vi "Write Current.vi"(8 "error in":errorcluster, 10 "Current":dbl, 11 "69X_79X in":refnum<class "79XRP.lvclass">) -> (0 "error out":errorcluster, 3 "69X_79X out":refnum<class "79XRP.lvclass">)   [LabVIEW 2019, in "79XRP.lvlib" / "79XRP.lvclass"]
uses:
  Library/79XRP.lvclass
  C:/Users/Public/Documents/Development/builds/Instruments/PowerSupply.lvlibp/Library/PowerSupply.lvclass
  Library/79XRP.lvclass/79XRP.ctl
  Read Local Resource.vi
  builds/Instruments/PowerSupply.lvlibp/Library/PowerSupply.lvclass
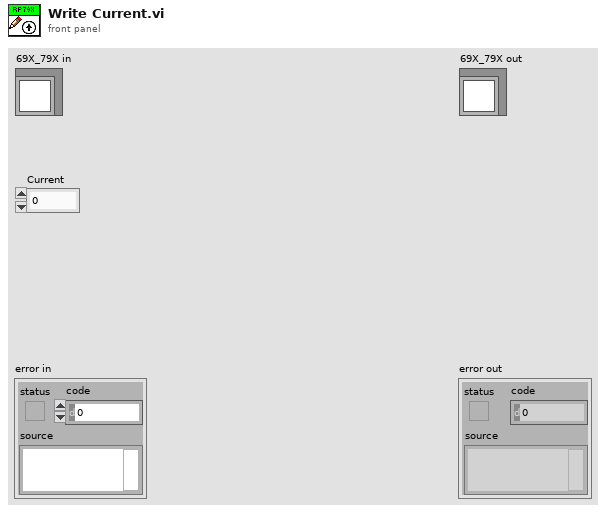
[diagram p1: front panel]
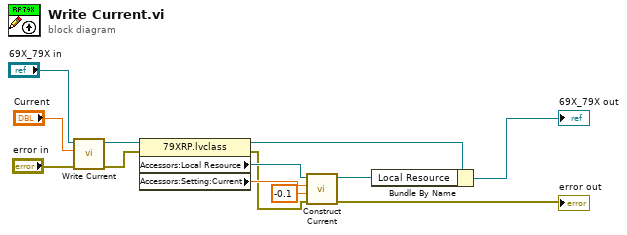
[diagram p0: block diagram]
diagram:
  n1 = call-parent "Write Current.vi"("error in"="error in", "Current"="Current", "PowerSupply in"="69X_79X in") -> ("error out"=w8:errorcluster, "PowerSupply out"=w10:refnum<class "79XRP.lvclass">)  [unwired: 7 in]
  n2 = property class="79XRP.lvclass"(reference=w10, error in=w8) -> (reference out=w9:refnum<class "79XRP.lvclass">, error out=w3:errorcluster, "Accessors:Local Resource"=w6:refnum<visa-resource-name>, "Accessors:Setting:Current"=w5:dbl)
  n3 = call "Construct Current.vi"("error in (no error)"=w3, "Negative Current Limit"=-0.1, "Positive Current Limit"=w5, "VISA resource name"=w6) -> ("error out"=→"error out":errorcluster, "VISA resource name out"=w2:refnum<visa-resource-name>)  [unwired: 6 in]
  n4 = Bundle By Name(cluster=w9, "Local Resource"=w2) -> (→"69X_79X out":refnum<class "79XRP.lvclass">)
